vi "Analysis.Build List of Unique Items, Str.vi"(10 "Item In":string, 11 "List In":string[](array[string])) -> (2 "Added":bool, 3 "List Out":string[](array[string]), 5 "Index":i32)   [LabVIEW 2024]
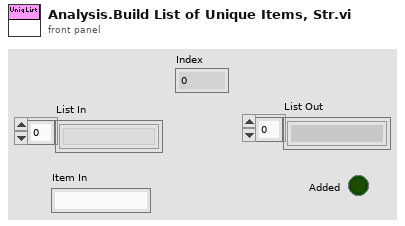
[diagram p1: front panel]
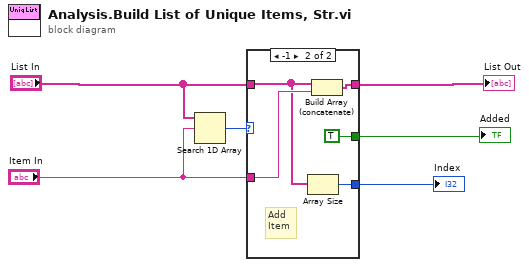
[diagram p0: block diagram]
diagram:
  n1 = Search 1D Array(1D array="List In", element="Item In") -> (index of element=w3:i32)  [unwired: 1 in]
  n2 = case shown="-1" w3 {
    selector: w3 -> [w7 _]
    tunnel: "Item In" -> [_ w12]
    tunnel: "List In" -> [w8 w9]
    tunnel: [w8 w13] -> w5
    tunnel: [_ TRUE] -> w2
    tunnel: [w7 w10] -> w1
    frame Default {
      # "Skip"
    }
    frame -1 {
      # "Add\nItem"
      n3 = Array Size(array=w9) -> (size(s)=w10:i32)
      n4 = Build Array (concatenate)(w9, w12) -> (w13:string[])
    }
  }
  "List Out" <- w5
  "Added" <- w2
  "Index" <- w1
